vi "orderbook.test.runner.vi"() -> ()   [LabVIEW 2020]
panel:
  out "Passed 4":bool
  in  "error in":errorcluster
  out "error out":errorcluster
  out "Passed 3":bool
  out "Passed 2":bool
  out "Passed":bool
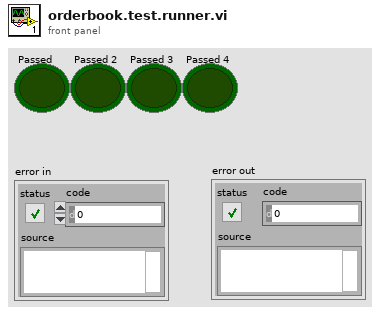
[diagram p1: front panel]
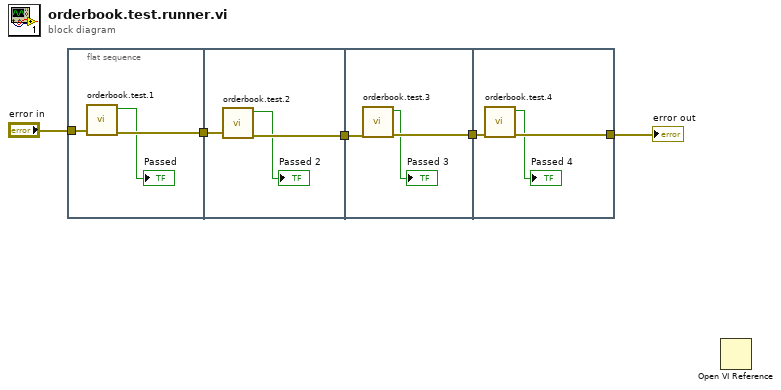
[diagram p0: block diagram]
diagram:
  n1 = flat-sequence {
    tunnel: [w8] -> w5
    tunnel: "error in" -> [w7]
    tunnel: w5 -> [w11]
    tunnel: [w10] -> w4
    tunnel: w4 -> [w14]
    tunnel: [w13] -> w1
    tunnel: [w16] -> w3
    tunnel: w1 -> [w17]
    frame #0 {
      n2 = call "orderbook.test.1.vi"("error in"=w7) -> ("error out"=w8:errorcluster, "Passed"=→"Passed":bool)  [unwired: 9 in]
    }
    frame #1 {
      n3 = call "orderbook.test.2.vi"("error in"=w11) -> ("error out"=w10:errorcluster, "Passed"=→"Passed 2":bool)  [unwired: 9 in]
    }
    frame #2 {
      n4 = call "orderbook.test.3.vi"("error in"=w14) -> ("error out"=w13:errorcluster, "Passed"=→"Passed 3":bool)  [unwired: 9 in]
    }
    frame #3 {
      n5 = call "orderbook.test.4.vi"("error in"=w17) -> ("error out"=w16:errorcluster, "Passed"=→"Passed 4":bool)  [unwired: 9 in]
    }
  }
  n6 = Open VI Reference() -> ()  [unwired: 6 in, 2 out]
  "error out" <- w3
